vi "Multi-Channel ADC.vi"(11 "error in":errorcluster) -> (15 "error out":errorcluster)   [LabVIEW 2023, in "Conversion.lvclass"]
doc: "This ADC converter VI converts the analog data to digital in two cases - Single channel where one analog data is converted to digital data, Multichannel where 4 input analog data is converted into digital data in 4 different channels."
uses:
  Classes/Conversion/Conversion.lvclass
  Type def/QueueOperations.ctl
  Type def/ADCData.ctl
  Type def/ADCType.ctl
  Type def/ChannelType.ctl
  Type def/Resolution.ctl
  Type def/U8ArrayCluster.ctl
  Type def/variant.ctl
panel:
  # "ANALOG TO DIGITAL CONVERSION  VI"
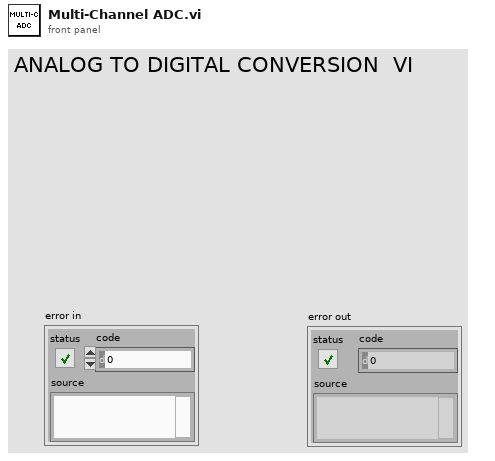
[diagram p1: front panel]
types:
  T1 = typedef "variant.ctl" = cluster{"Data":variant, "State":string}
  T2 = typedef "ADCData.ctl" = cluster{"Start time":dbl, "Sampling rate":dbl, "Start":bool, "ADC Type":T3, "Conversion Class":refnum<class "Conversion.lvclass">, "Single Channel class":refnum<class "Conversion.lvclass">, "Multi Channel class":refnum<class "Conversion.lvclass">, "Classes Path Array":path[], "U8 Array Cluster":T6, "Notifier Single":refnum<notifier>, "Notifier Multi":refnum<notifier>}
  T3 = typedef "ADCType.ctl" = cluster{"Channel Type":T4, "Resolution":T5}
  T4 = typedef "ChannelType.ctl" = enum16{"Single", "4-Channel"}
  T5 = typedef "Resolution.ctl" = enum16{"2", "4", "8", "12", "16"}
  T6 = typedef "U8ArrayCluster.ctl" = cluster{"Single Channel U8 array":u8[], "Mult Channel U8 array":u8[][], "1D Multi Channel U8 Array":u8[], "Channel 1 U8 Array":u8[], "Channel 2 U8 Array":u8[], "Channel 3 U8 Array":u8[], "Channel 4 U8 Array":u8[]}
  T7 = typedef "QueueOperations.ctl" = enum16{"Create", "Enqueue", "Enqueue N elements", "Dequeue", "Flush", "Release"}
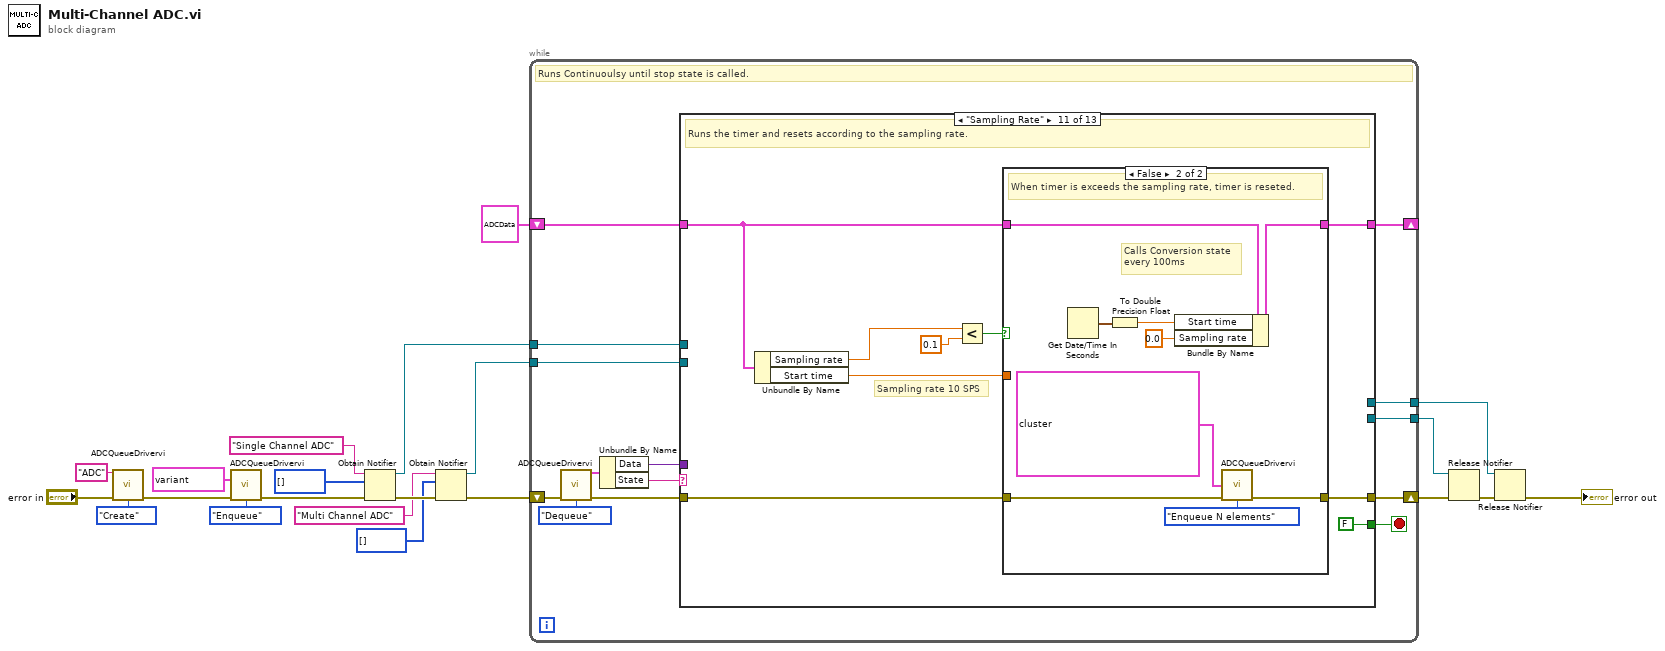
[diagram p0: block diagram]
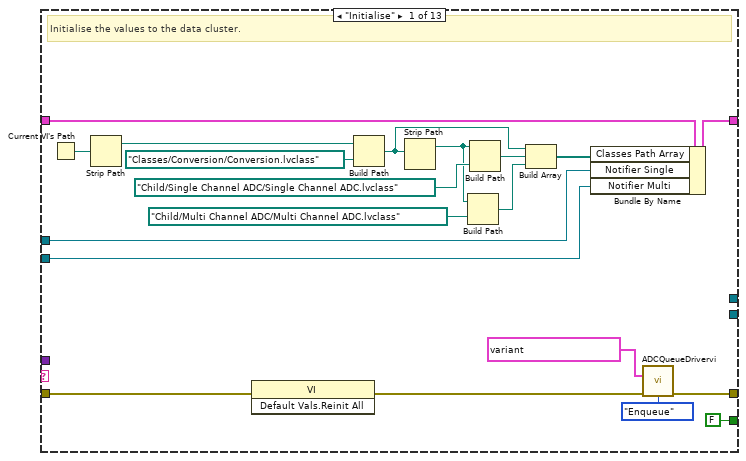
[diagram p2: hidden frame]
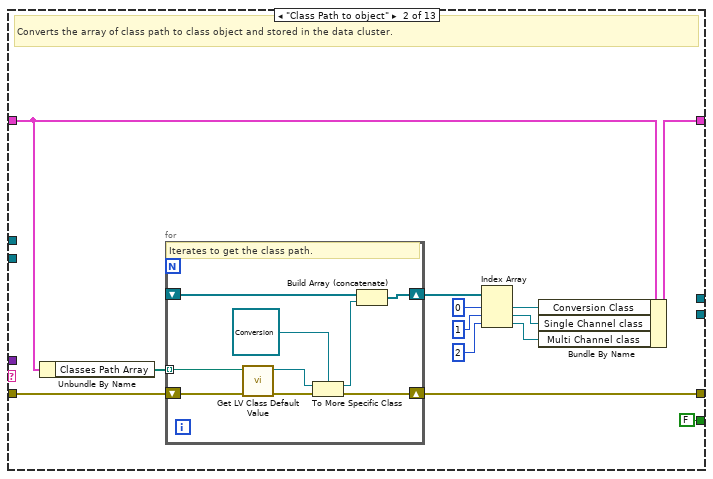
[diagram p3: hidden frame]
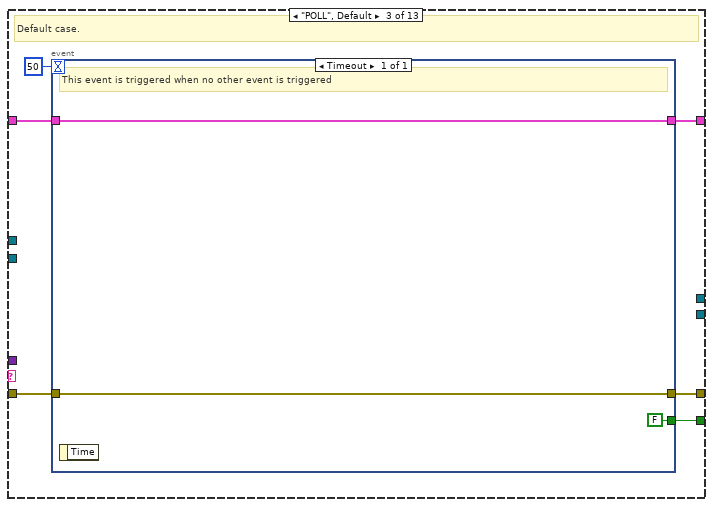
[diagram p4: hidden frame]
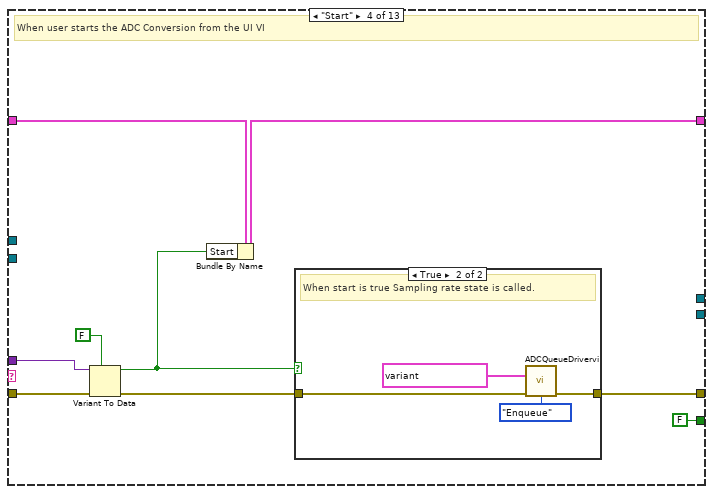
[diagram p5: hidden frame]
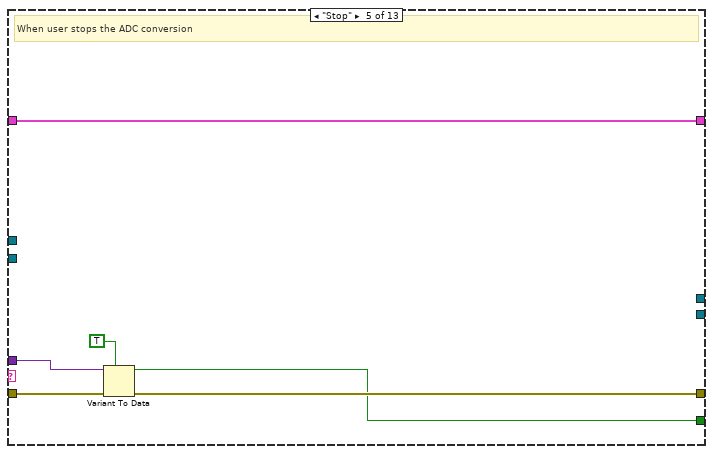
[diagram p7: hidden frame]
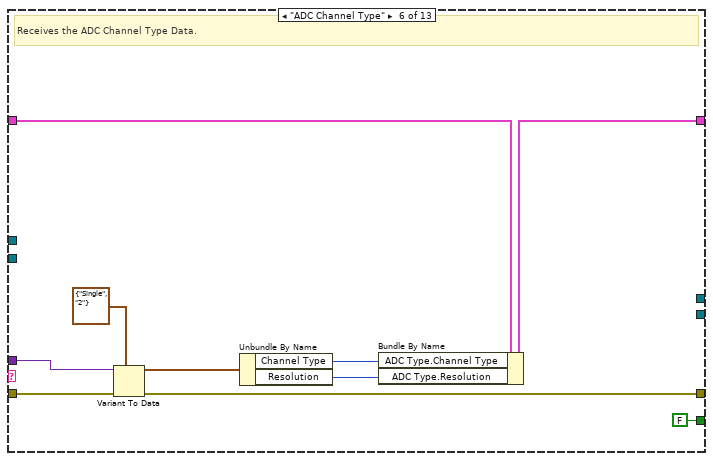
[diagram p8: hidden frame]
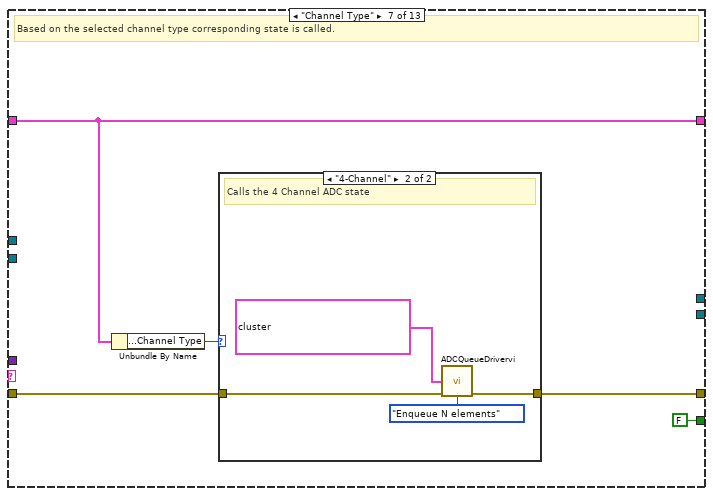
[diagram p9: hidden frame]
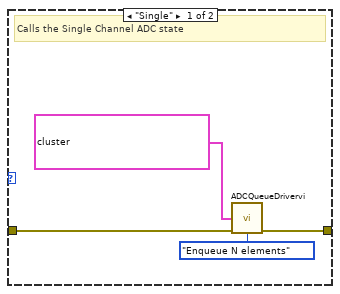
[diagram p10: hidden frame]
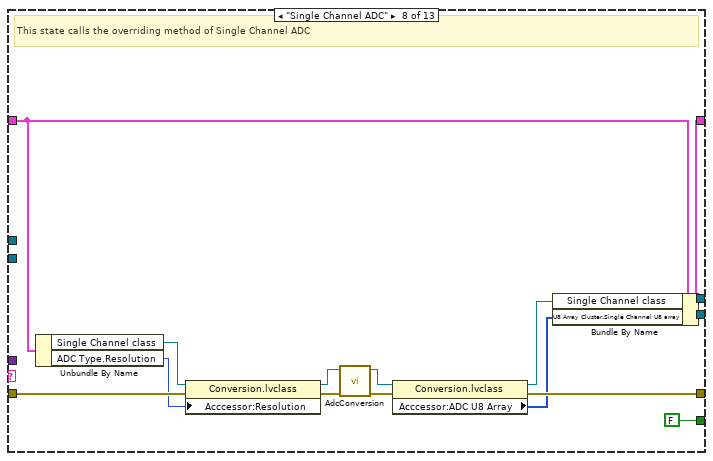
[diagram p11: hidden frame]
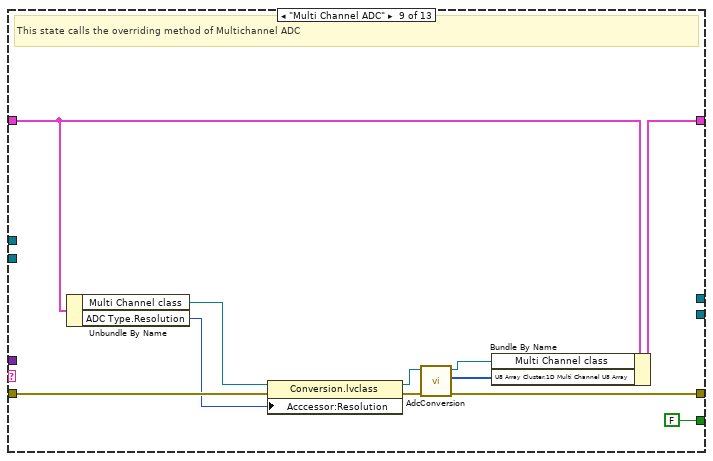
[diagram p12: hidden frame]
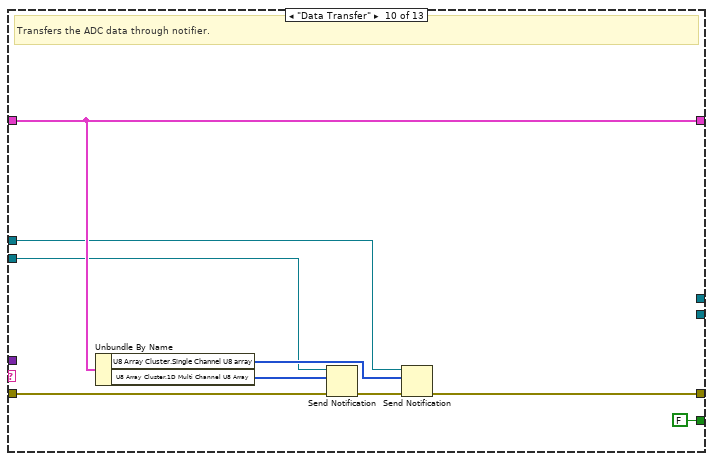
[diagram p13: hidden frame]
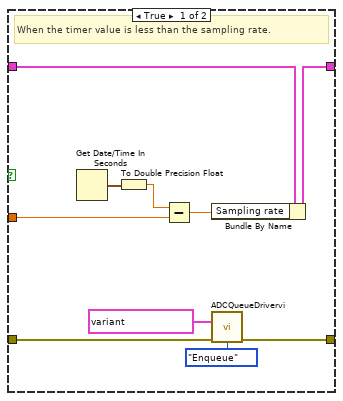
[diagram p14: hidden frame]
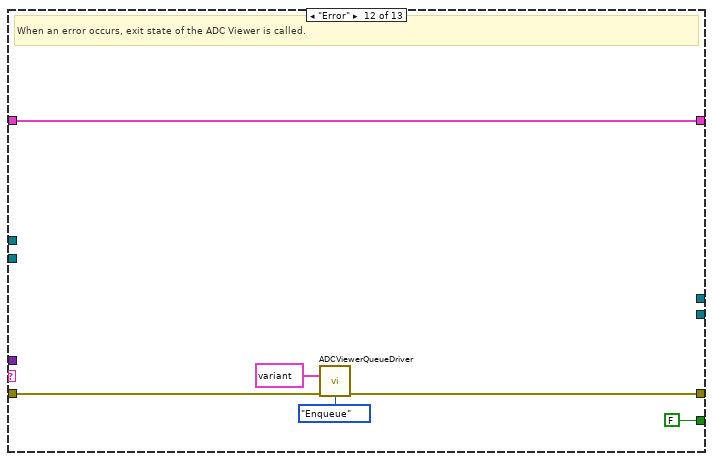
[diagram p15: hidden frame]
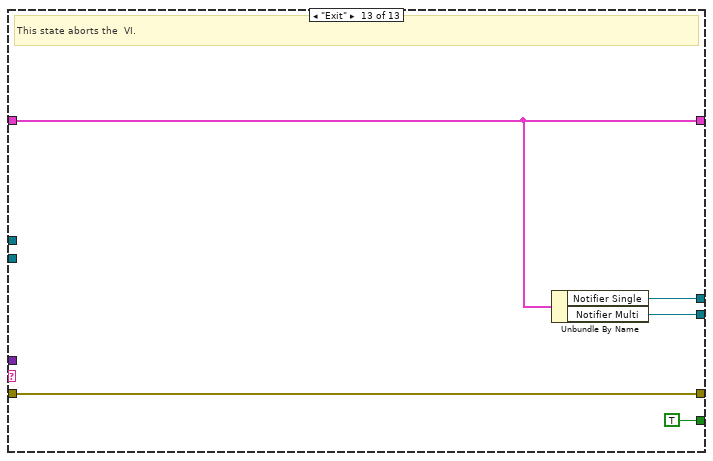
[diagram p16: hidden frame]
diagram:
  n1 = call "ADCQueueDrivervi.vi"("Queue Name"="ADC", "error in"="error in", "Queue Operations"=QueueOperations."Create") -> ("error out"=w20:errorcluster)  [unwired: 11 in, 1 out]
  n2 = call "ADCQueueDrivervi.vi"("Enqueue State"=T1 {"Data"=variant, "State"="Initialise"}, "error in"=w20, "Queue Operations"=QueueOperations."Enqueue") -> ("error out"=w13:errorcluster)  [unwired: 11 in, 1 out]
  n3 = Obtain Notifier(name (unnamed)="Single Channel ADC", notification data type=u8[] [] ("appended array"), error in (no error)=w13) -> (notifier out=w12:refnum<notifier>, error out=w10:errorcluster)  [unwired: 1 in, 1 out]
  n4 = Obtain Notifier(name (unnamed)="Multi Channel ADC", notification data type=u8[] [] ("1D Multi Channnel Array"), error in (no error)=w10) -> (notifier out=w6:refnum<notifier>, error out=w9:errorcluster)  [unwired: 1 in, 1 out]
  n5 = while {
    shift-right: [w30] -> w5
    shift-left: w9 -> [w34]
    shift-right: [w27] -> _
    shift-left: T2 {"Start time"=0.0, "Sampling rate"=0.0, "Start"=FALSE, "ADC Type"={"Channel Type"=enum."Single", "Resolution"=enum."2"}, "Conversion Class"=refnum, "Single Channel class"=refnum, "Multi Channel class"=refnum, "Classes Path Array"=[], "U8 Array Cluster"={"Single Channel U8 array"=[], "Mult Channel U8 array"=[], "1D Multi Channel U8 Array"=[], "Channel 1 U8 Array"=[], "Channel 2 U8 Array"=[], "Channel 3 U8 Array"=[], "Channel 4 U8 Array"=[]}, "Notifier Single"=refnum, "Notifier Multi"=refnum} -> [w28]
    tunnel: w12 -> [w26]
    tunnel: w6 -> [w25]
    tunnel: [w23] -> w2
    tunnel: [w22] -> w1
    stop <- w29 stop-if-true
    # "Runs Continuoulsy until stop state is called."
    n6 = call "ADCQueueDrivervi.vi"("error in"=w34, "Queue Operations"=QueueOperations."Dequeue") -> ("Dequeue State"=w32:T1, "error out"=w33:errorcluster)  [unwired: 12 in]
    n7 = Unbundle By Name(w32) -> ("Data"=w31:variant, "State"=w24:string)
    n8 = case shown="\"Sampling Rate\"" w24 {
      tunnel: w33 -> [w54 w57 w82 w95 w105 w116 w119 w139 w150 w157 w168 w193 w200]
      tunnel: w31 -> [_ _ _ w92 w103 w109 _ _ _ _ _ _ _]
      tunnel: [w49 w56 w81 w88 w104 w113 w118 w133 w145 w159 w167 w192 w200] -> w30
      tunnel: [FALSE FALSE ("Discard?") w83 FALSE ("Discard?") w101 FALSE ("Discard?") FALSE ("Discard?") FALSE FALSE FALSE ("Discard?") FALSE FALSE TRUE] -> w29
      tunnel: w28 -> [w52 w67 w80 w94 w106 w115 w120 w141 w152 w161 w170 w196 w199]
      tunnel: [w51 w61 w79 w91 w106 w112 w120 w140 w151 w161 w169 w196 w199] -> w27
      tunnel: w26 -> [w37 _ _ _ _ _ _ _ _ w158 _ _ _]
      tunnel: w25 -> [w36 _ _ _ _ _ _ _ _ w155 _ _ _]
      tunnel: [_ _ _ _ _ _ _ _ _ _ _ _ w198] -> w23
      tunnel: [_ _ _ _ _ _ _ _ _ _ _ _ w197] -> w22
      frame "Initialise" {
        # "Initialise the values to the data cluster."
        n9 = Current VI's Path() -> (path=w47:path)
        n10 = Strip Path(path=w47) -> (stripped path=w46:path)  [unwired: 1 out]
        n11 = invoke class="VI" method="Default Vals.Reinit All"(error in=w54) -> (error out=w53:errorcluster)  [unwired: 2 in, 2 out]
        n12 = Build Path(base path=w46, name or relative path=path "Classes/Conversion/Conversion.lvclass") -> (appended path=w43:path)
        n13 = Strip Path(path=w43) -> (stripped path=w41:path)  [unwired: 1 out]
        n14 = Build Path(base path=w41, name or relative path=path "Child/Multi Channel ADC/Multi Channel ADC.lvclass") -> (appended path=w39:path)
        n15 = Build Path(base path=w41, name or relative path=path "Child/Single Channel ADC/Single Channel ADC.lvclass") -> (appended path=w40:path)
        n16 = Build Array(w43, w40, w39) -> (w38:path[])
        n17 = Bundle By Name(cluster=w52, "Classes Path Array"=w38, "Notifier Single"=w37, "Notifier Multi"=w36) -> (w51:T2)
        n18 = call "ADCQueueDrivervi.vi"("Enqueue State"=T1 {"Data"=variant, "State"="Class Path to object"}, "error in"=w53, "Queue Operations"=QueueOperations."Enqueue") -> ("error out"=w49:errorcluster)  [unwired: 11 in, 1 out]
      }
      frame "Class Path to object" {
        # "Converts the array of class path to class object and stored in the data cluster."
        n19 = Unbundle By Name(w67) -> ("Classes Path Array"=w66:path[])
        n20 = for {
          tunnel: w66 -> [w74] mode=indexing
          shift-right: [w73] -> w56
          shift-left: w57 -> [w72]
          shift-right: [w70] -> w65
          shift-left: _ -> [w69]
          # "Iterates to get the class path."
          n21 = call <vilib>:"Get LV Class Default Value.vi"("error in (no error)"=w72, "class path"=w74) -> ("error out"=w77:errorcluster, "object"=w76:refnum<class>)  [unwired: 8 in]
          n22 = To More Specific Class(target class=refnum<class "Conversion.lvclass"> refnum ("Conversion.lvclass"), reference=w76, error in=w77) -> (specific class reference=w71:refnum<class "Conversion.lvclass">, error out=w73:errorcluster)
          n23 = Build Array (concatenate)(w69, w71) -> (w70:refnum<class "Conversion.lvclass">[])
        }
        n24 = Index Array(array=w65, index #1=0 ("index"), index #2=1 ("index"), index #3=2 ("index")) -> (element #1=w60:refnum<class "Conversion.lvclass">, element #2=w59:refnum<class "Conversion.lvclass">, element #3=w58:refnum<class "Conversion.lvclass">)
        n25 = Bundle By Name(cluster=w67, "Conversion Class"=w60, "Single Channel class"=w59, "Multi Channel class"=w58) -> (w61:T2)
      }
      frame "POLL", Default {
        # "Default case."
        n26 = event shown="[0] Timeout" {
          selector: _ -> [_]
          dyn-events: _ -> [_]
          timeout: 50 -> [_]
          tunnel: [FALSE ("Discard?")] -> w83
          tunnel: w82 -> [w85]
          tunnel: [w85] -> w81
          tunnel: w80 -> [w84]
          tunnel: [w84] -> w79
          event Timeout {
            # "This event is triggered when no other event is triggered"
            n27 = event-data() -> ()  [unwired: 1 in, 1 out]
          }
        }
      }
      frame "Start" {
        # "When user starts the ADC Conversion from the UI VI"
        n28 = Variant To Data(error in=w95, type=FALSE ("Start"), Variant=w92) -> (data=w87:bool, error out=w89:errorcluster)
        n29 = Bundle By Name(cluster=w94, "Start"=w87) -> (w91:T2)
        n30 = case shown="True" w87 {
          tunnel: w89 -> [w96 w98]
          tunnel: [w96 w97] -> w88
          frame False {
            # "When start is false."
          }
          frame True {
            # "When start is true Sampling rate state is called."
            n31 = call "ADCQueueDrivervi.vi"("Enqueue State"=T1 {"Data"=variant, "State"="Sampling Rate"}, "error in"=w98, "Queue Operations"=QueueOperations."Enqueue") -> ("error out"=w97:errorcluster)  [unwired: 11 in, 1 out]
          }
        }
      }
      frame "Stop" {
        # "When user stops the ADC conversion"
        n32 = Variant To Data(error in=w105, type=TRUE, Variant=w103) -> (data=w101:bool, error out=w104:errorcluster)
      }
      frame "ADC Channel Type" {
        # "Receives the ADC Channel Type Data."
        n33 = Variant To Data(error in=w116, type=T3 {"Channel Type"=enum."Single", "Resolution"=enum."2"} ("input cluster"), Variant=w109) -> (data=w107:T3, error out=w113:errorcluster)
        n34 = Unbundle By Name(w107) -> ("Channel Type"=w111:T4, "Resolution"=w110:T5)
        n35 = Bundle By Name(cluster=w115, "ADC Type.Channel Type"=w111, "ADC Type.Resolution"=w110) -> (w112:T2)
      }
      frame "Channel Type" {
        # "Based on the selected channel type corresponding state is called."
        n36 = Unbundle By Name(w120) -> ("ADC Type.Channel Type"=w117:T4)
        n37 = case shown="\"4-Channel\"" w117 {
          tunnel: w119 -> [w123 w127]
          tunnel: [w122 w126] -> w118
          frame "Single" {
            # "Calls the Single Channel ADC state"
            n38 = call "ADCQueueDrivervi.vi"("Array State"=T1[] [{"Data"=variant, "State"="Single Channel ADC"}], "error in"=w123, "Queue Operations"=QueueOperations."Enqueue N elements") -> ("error out"=w122:errorcluster)  [unwired: 11 in, 1 out]
          }
          frame "4-Channel" {
            # "Calls the 4 Channel ADC state"
            n39 = call "ADCQueueDrivervi.vi"("Array State"=T1[] [{"Data"=variant, "State"="Multi Channel ADC"}], "error in"=w127, "Queue Operations"=QueueOperations."Enqueue N elements") -> ("error out"=w126:errorcluster)  [unwired: 11 in, 1 out]
          }
        }
      }
      frame "Single Channel ADC" {
        # "This state calls the overriding method of Single Channel ADC"
        n40 = Unbundle By Name(w141) -> ("Single Channel class"=w136:refnum<class "Conversion.lvclass">, "ADC Type.Resolution"=w135:T5)
        n41 = property class="Conversion.lvclass"(reference=w136, error in=w139, "Acccessor:Resolution"=w135) -> (reference out=w134:refnum<class "Conversion.lvclass">, error out=w137:errorcluster)
        n42 = call-dynamic "AdcConversion.vi"("error in (no error)"=w137, "Conversion in"=w134) -> ("error out"=w138:errorcluster, "Conversion out"=w132:refnum<class "Conversion.lvclass">)  [unwired: 7 in, 1 out]
        n43 = property class="Conversion.lvclass"(reference=w132, error in=w138) -> (reference out=w130:refnum<class "Conversion.lvclass">, error out=w133:errorcluster, "Acccessor:ADC U8 Array"=w131:u8[])
        n44 = Bundle By Name(cluster=w141, "Single Channel class"=w130, "U8 Array Cluster.Single Channel U8 array"=w131) -> (w140:T2)
      }
      frame "Multi Channel ADC" {
        # "This state calls the overriding method of Multichannel ADC"
        n45 = Unbundle By Name(w152) -> ("Multi Channel class"=w148:refnum<class "Conversion.lvclass">, "ADC Type.Resolution"=w147:T5)
        n46 = property class="Conversion.lvclass"(reference=w148, error in=w150, "Acccessor:Resolution"=w147) -> (reference out=w146:refnum<class "Conversion.lvclass">, error out=w149:errorcluster)
        n47 = call-dynamic "AdcConversion.vi"("error in (no error)"=w149, "Conversion in"=w146) -> ("error out"=w145:errorcluster, "ADC U8 Array"=w143:u8[], "Conversion out"=w144:refnum<class "Conversion.lvclass">)  [unwired: 7 in]
        n48 = Bundle By Name(cluster=w152, "Multi Channel class"=w144, "U8 Array Cluster.1D Multi Channel U8 Array"=w143) -> (w151:T2)
      }
      frame "Data Transfer" {
        # "Transfers the ADC data through notifier."
        n49 = Unbundle By Name(w161) -> ("U8 Array Cluster.Single Channel U8 array"=w160:u8[], "U8 Array Cluster.1D Multi Channel U8 Array"=w154:u8[])
        n50 = Send Notification(notification=w154, notifier=w155, error in (no error)=w157) -> (error out=w156:errorcluster)  [unwired: 1 out]
        n51 = Send Notification(notification=w160, notifier=w158, error in (no error)=w156) -> (error out=w159:errorcluster)  [unwired: 1 out]
      }
      frame "Sampling Rate" {
        # "Sampling rate 10 SPS"
        # "Runs the timer and resets according to the sampling rate."
        n52 = Unbundle By Name(w170) -> ("Sampling rate"=w165:dbl, "Start time"=w166:dbl)
        n53 = Less?(x=w165, y=0.1) -> (x < y?=w163:bool)
        n54 = case shown="False" w163 {
          tunnel: w170 -> [w181 w190]
          tunnel: [w179 w188] -> w169
          tunnel: w168 -> [w175 w187]
          tunnel: [w174 w186] -> w167
          tunnel: w166 -> [w176 _]
          frame True {
            # "When the timer value is less than the sampling rate."
            n55 = Get Date/Time In Seconds() -> (seconds since 1Jan1904=w180:timestamp)
            n56 = To Double Precision Float(number=w180) -> (double precision float=w177:dbl)
            n57 = Subtract(x=w177, y=w176) -> (x-y=w178:dbl)
            n58 = Bundle By Name(cluster=w181, "Sampling rate"=w178) -> (w179:T2)
            n59 = call "ADCQueueDrivervi.vi"("Enqueue State"=T1 {"Data"=variant, "State"="Sampling Rate"}, "error in"=w175, "Queue Operations"=QueueOperations."Enqueue") -> ("error out"=w174:errorcluster)  [unwired: 11 in, 1 out]
          }
          frame False {
            # "Calls Conversion state\nevery 100ms"
            # "When timer is exceeds the sampling rate, timer is reseted."
            n60 = Get Date/Time In Seconds() -> (seconds since 1Jan1904=w189:timestamp)
            n61 = To Double Precision Float(number=w189) -> (double precision float=w184:dbl)
            n62 = Bundle By Name(cluster=w190, "Start time"=w184, "Sampling rate"=0.0) -> (w188:T2)
            n63 = call "ADCQueueDrivervi.vi"("Array State"=T1[] [{"Data"=variant, "State"="Sampling Rate"}, {"Data"=variant, "State"="Channel Type"}, {"Data"=variant, "State"="Data Transfer"}], "error in"=w187, "Queue Operations"=QueueOperations."Enqueue N elements") -> ("error out"=w186:errorcluster)  [unwired: 11 in, 1 out]
          }
        }
      }
      frame "Error" {
        # "When an error occurs, exit state of the ADC Viewer is called."
        n64 = call "ADCViewerQueueDriver.vi"("Enqueue State"=T1 {"Data"=variant, "State"="Exit"}, "error in"=w193, "Queue Operations"=QueueOperations."Enqueue") -> ("error out"=w192:errorcluster)  [unwired: 11 in, 1 out]
      }
      frame "Exit" {
        # "This state aborts the  VI."
        n65 = Unbundle By Name(w199) -> ("Notifier Single"=w197:refnum<notifier>, "Notifier Multi"=w198:refnum<notifier>)
      }
    }
  }
  n66 = Release Notifier(notifier=w2, error in (no error)=w5) -> (error out=w4:errorcluster)  [unwired: 1 in, 2 out]
  n67 = Release Notifier(notifier=w1, error in (no error)=w4) -> (error out=→"error out":errorcluster)  [unwired: 1 in, 2 out]
